vi "eFGV - Modbus Reply.vi"(6 "State - eFGV":T3=enum."Close", 8 "error in (no error)":errorcluster, 10 "Modbus Reply":T1) -> (0 "error out":errorcluster, 2 "Event - Modbus Reply":refnum<user-event>)   [LabVIEW 2020]
uses:
  Control/State - eFGV.ctl
  Control/Data Struct - Modbus Reply.ctl
  Control/Device Name.ctl
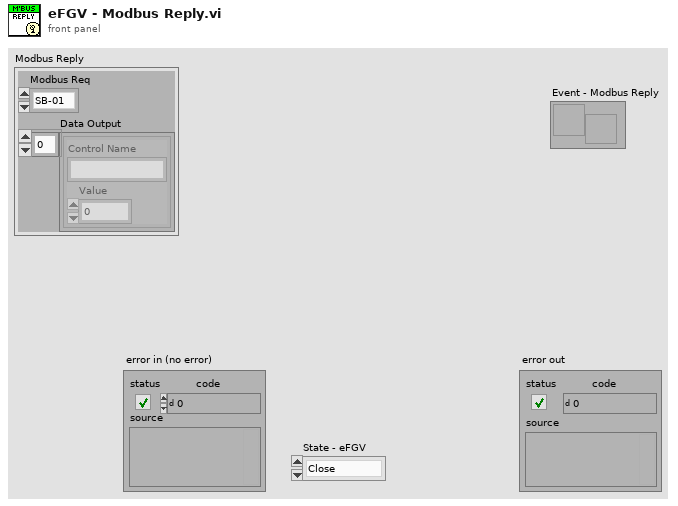
[diagram p1: front panel]
types:
  T1 = typedef "Data Struct - Modbus Reply.ctl" = cluster{"Modbus Req":T2, "Data Output":cluster{"Control Name":string, "Value":dbl}[]}
  T2 = typedef "Device Name.ctl" = enum16{"SB-01", "SB-02", "BANK-01", "BANK-02", "SI-M", "SI-S01", "SI-S02", "PM-01"}
  T3 = typedef "State - eFGV.ctl" = enum16{"Init", "Read", "Write", "Close"}
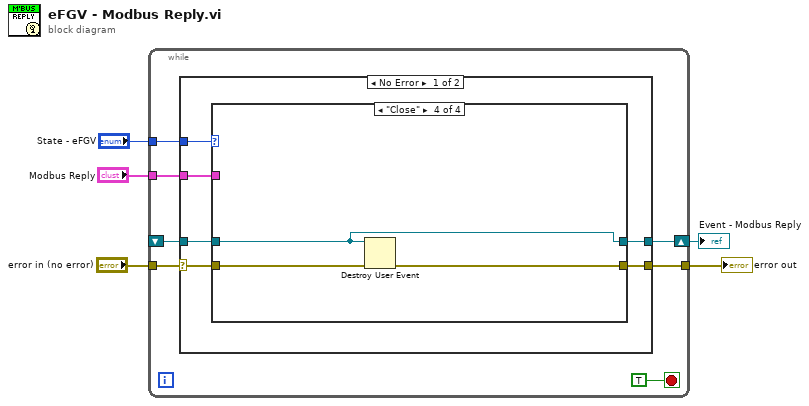
[diagram p0: block diagram]
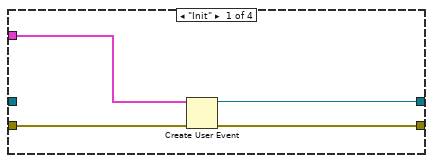
[diagram p2: hidden frame]
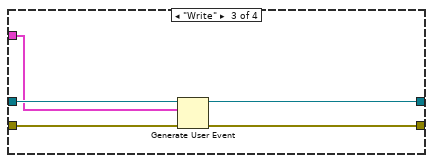
[diagram p4: hidden frame]
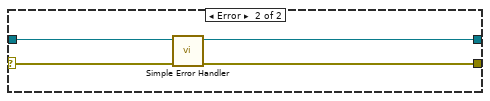
[diagram p5: hidden frame]
diagram:
  n1 = while {
    tunnel: "State - eFGV" -> [w11]
    tunnel: "error in (no error)" -> [w10]
    tunnel: [w9] -> w3
    shift-right: [w8] -> w1
    shift-left: _ -> [w7]
    tunnel: "Modbus Reply" -> [w6]
    stop <- TRUE stop-if-true
    n2 = case shown="No Error" w10 {
      selector: w10 -> [w17 w35]
      tunnel: w11 -> [w18 _]
      tunnel: [w16 w33] -> w9
      tunnel: [w15 w34] -> w8
      tunnel: w7 -> [w14 w34]
      tunnel: w6 -> [w13 _]
      frame No Error {
        n3 = case shown="\"Close\"" w18 {
          tunnel: w17 -> [w22 w24 w29 w32]
          tunnel: [w21 w24 w28 w31] -> w16
          tunnel: [w20 w23 w27 w30] -> w15
          tunnel: w14 -> [_ w23 w26 w30]
          tunnel: w13 -> [w19 _ w25 _]
          frame "Init" {
            n4 = Create User Event(user event datatype=w19, error in=w22) -> (user event=w20:refnum<user-event>, error out=w21:errorcluster)
          }
          frame "Read", Default {
          }
          frame "Write" {
            n5 = Generate User Event(user event=w26, event data cluster=w25, error in=w29) -> (user event out=w27:refnum<user-event>, error out=w28:errorcluster)  [unwired: 1 in]
          }
          frame "Close" {
            n6 = Destroy User Event(user event=w30, error in=w32) -> (error out=w31:errorcluster)
          }
        }
      }
      frame Error {
        n7 = call <vilib>:"Simple Error Handler.vi"("error in (no error)"=w35) -> ("error out"=w33:errorcluster)  [unwired: 4 in, 4 out]
      }
    }
  }
  "error out" <- w3
  "Event - Modbus Reply" <- w1
